vi "Decode UDP Message_2.vi"(11 "Input string":string) -> (3 "Data":T1={"Command"=enum."Speed", "Msg Length"=0, "Content Bytes"=[], "Content String"="", "CRC8"=0, "Valid?"=FALSE})   [LabVIEW 2015]
uses:
  controls/UDP Message Data.ctl
  <vilib>/regexp/Match Regular Expression.xnode
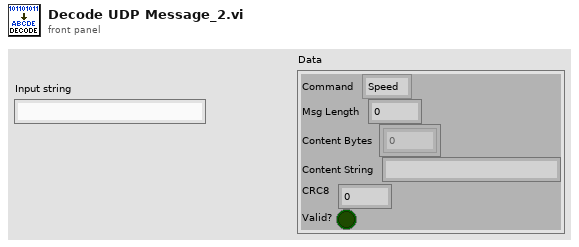
[diagram p1: front panel]
types:
  T1 = typedef "UDP Message Data.ctl" = cluster{"Command":enum16{"Acknowledge", "Speed", "Brake", "Watchdog", "Update", "Exit", "Init", "Log", "Unknown"}, "Msg Length":u8, "Content Bytes":u8[], "Content String":string, "CRC8":u8, "Valid?":bool}
  T2 = enum16{"Acknowledge", "Speed", "Brake", "Watchdog", "Update", "Exit", "Init", "Log", "Unknown"}
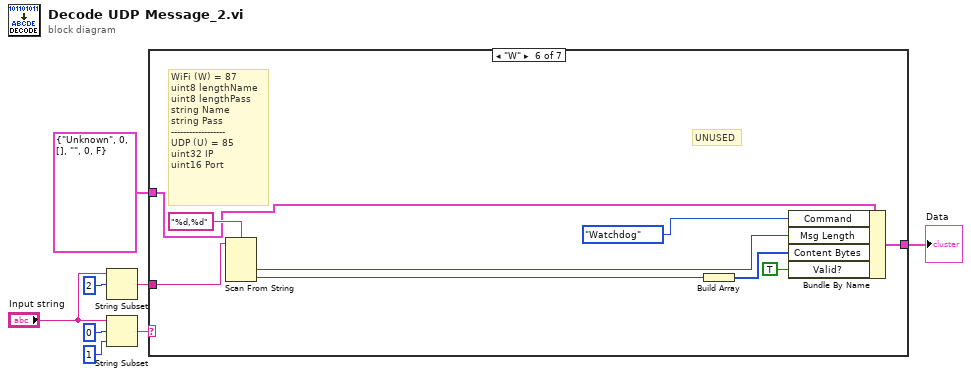
[diagram p0: block diagram]
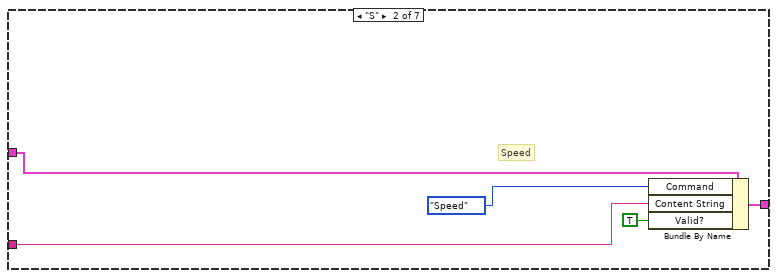
[diagram p3: hidden frame]
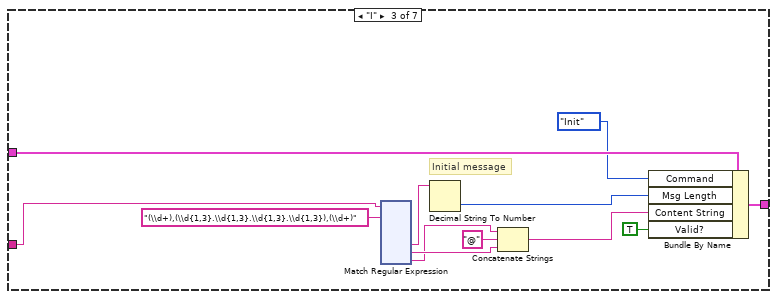
[diagram p4: hidden frame]
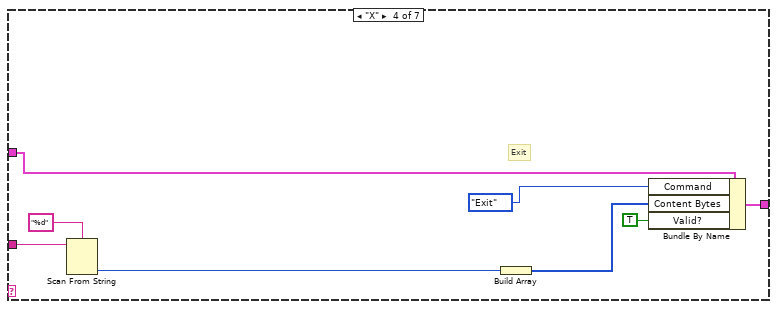
[diagram p5: hidden frame]
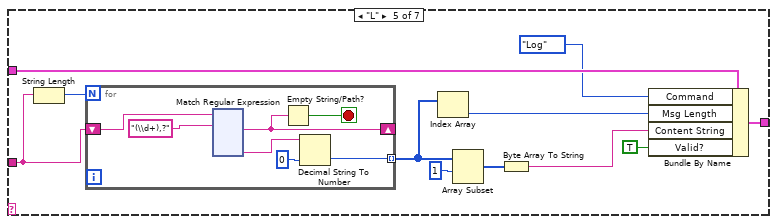
[diagram p6: hidden frame]
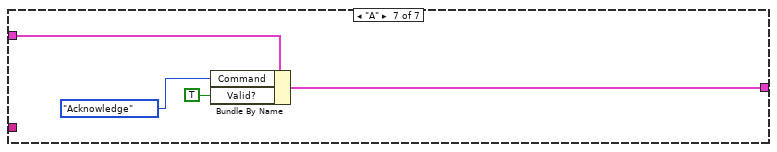
[diagram p7: hidden frame]
diagram:
  n1 = String Subset(string="Input string", offset (0)=2) -> (substring=w4:string)  [unwired: 1 in]
  n2 = String Subset(string="Input string", offset (0)=0, length (rest)=1 ("length (rest)")) -> (substring=w7:string)
  n3 = case shown="\"W\"" w7 {
    tunnel: w4 -> [_ w11 w22 w151 w159 w294 _]
    tunnel: T1 {"Command"=enum."Unknown", "Msg Length"=0, "Content Bytes"=[], "Content String"="", "CRC8"=0, "Valid?"=FALSE} ("Data") -> [w9 w14 w26 w150 w163 w293 w299]
    tunnel: [w9 w12 w25 w148 w160 w290 w297] -> w2
    frame Default {
    }
    frame "S" {
      # "Speed"
      n4 = Bundle By Name(cluster=w14, "Command"=T2."Speed", "Content String"=w11, "Valid?"=TRUE) -> (w12:T1)
    }
    frame "I" {
      # "Initial message"
      n5 = xnode "Match Regular Expression"("input string"=w22, "regular expression"="(\\d+),(\\d{1,3}.\\d{1,3}.\\d{1,3}.\\d{1,3}),(\\d+)") -> ("submatch 1"=w21:string, "submatch 2"=w17:string, "submatch 3"=w16:string)  [unwired: 4 in, 5 out]
      n6 = Decimal String To Number(string=w21) -> (number=w20:i32)  [unwired: 2 in, 1 out]
      n7 = Concatenate Strings(w16, "@" ("input 2"), w17) -> (w18:string)
      n8 = Bundle By Name(cluster=w26, "Command"=T2."Init", "Msg Length"=w20, "Content String"=w18, "Valid?"=TRUE) -> (w25:T1)
    }
    frame "X" {
      # "Exit"
      n9 = Scan From String(format string="%d", input string=w151) -> (output 1=w147:i32)  [unwired: 3 in, 3 out]
      n10 = Build Array(w147) -> (w146:i32[])
      n11 = Bundle By Name(cluster=w150, "Command"=T2."Exit", "Content Bytes"=w146, "Valid?"=TRUE) -> (w148:T1)
    }
    frame "L" {
      n12 = String Length(string=w159) -> (length=w158:i32)
      n13 = for {
        N: w158 -> [_]
        shift-right: [w165] -> _
        shift-left: w159 -> [w170]
        tunnel: [w166] -> w155 mode=indexing
        stop <- w164 stop-if-true
        n14 = xnode "Match Regular Expression"("input string"=w170, "regular expression"="(\\d+),?") -> ("after match"=w165:string, "submatch 1"=w168:string)  [unwired: 4 in, 4 out]
        n15 = Empty String/Path?(string/path=w165) -> (empty?=w164:bool)
        n16 = Decimal String To Number(string=w168, default (0L)=u8 0 ("default (0 I32)")) -> (number=w166:u8)  [unwired: 1 in, 1 out]
      }
      n17 = Index Array(array=w155) -> (element=w154:u8)  [unwired: 1 in]
      n18 = Array Subset(array=w155, index=1) -> (w157:u8[])  [unwired: 1 in]
      n19 = Byte Array To String(unsigned byte array=w157) -> (string=w162:string)
      n20 = Bundle By Name(cluster=w163, "Command"=T2."Log", "Msg Length"=w154, "Content String"=w162, "Valid?"=TRUE) -> (w160:T1)
    }
    frame "W" {
      # "UNUSED"
      # "WiFi (W) = 87\nuint8 lengthName\nuint8 lengthPass\nstring Name\nstring Pass\n------------------\nUDP (U) = 85\nuint32 IP\nuint16 Port"
      n21 = Scan From String(format string="%d,%d", input string=w294) -> (output 1=w292:i32, output 2=w289:i32)  [unwired: 4 in, 3 out]
      n22 = Build Array(w289) -> (w288:i32[])
      n23 = Bundle By Name(cluster=w293, "Command"=T2."Watchdog", "Msg Length"=w292, "Content Bytes"=w288, "Valid?"=TRUE) -> (w290:T1)
    }
    frame "A" {
      n24 = Bundle By Name(cluster=w299, "Command"=T2."Acknowledge", "Valid?"=TRUE) -> (w297:T1)
    }
  }
  "Data" <- w2
